vi "http_redirect.vi"(10 "Value":string, 11 "HTTP Request in in":T1) -> (3 "HTTP Request in out":T1)   [LabVIEW 2011]
uses:
  http_request_response.ctl
  http_request.ctl
  http_field.ctl
  http_response.ctl
  template_field.ctl
  template_field_type.ctl
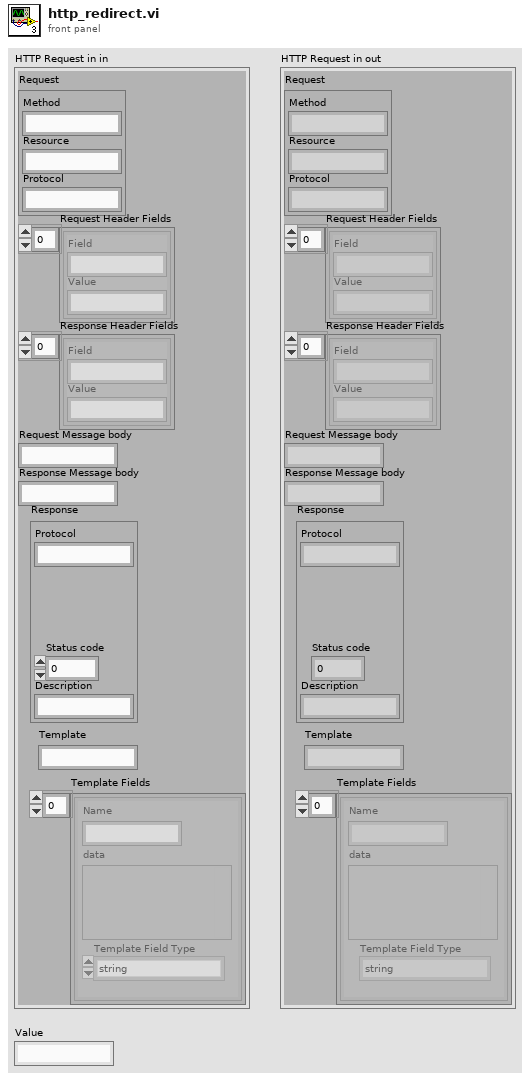
[diagram p1: front panel]
types:
  T1 = typedef "http_request_response.ctl" = cluster{"Request":T2, "Request Header Fields":T3[], "Response Header Fields":T3[], "Request Message body":string, "Response Message body":string, "Response":T4, "Template":string, "Template Fields":T5[]}
  T2 = typedef "http_request.ctl" = cluster{"Method":string, "Resource":string, "Protocol":string}
  T3 = typedef "http_field.ctl" = cluster{"Field":string, "Value":string}
  T4 = typedef "http_response.ctl" = cluster{"Protocol":string, "Status code":dbl, "Description":string}
  T5 = typedef "template_field.ctl" = cluster{"Name":string, "Template Field Type":T6, "data":variant}
  T6 = typedef "template_field_type.ctl" = enum16{"string", "string array", "number", "number array", "cluster", "cluster array"}
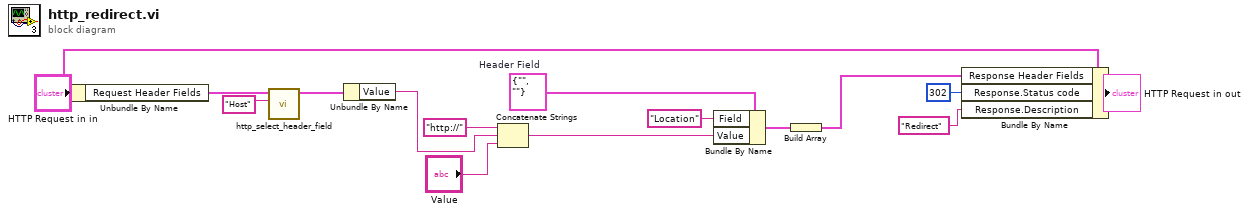
[diagram p0: block diagram]
diagram:
  w3 = T3 {"Field"="", "Value"=""}  # Header Field
  n1 = Unbundle By Name("HTTP Request in in") -> ("Request Header Fields"=w7:T3[])
  n2 = call "http_select_header_field.vi"("Name"="Host", "Request Header Fields"=w7) -> ("Header Field"=w9:T3)  [unwired: 8 in, 1 out]
  n3 = Unbundle By Name(w9) -> ("Value"=w10:string)
  n4 = Concatenate Strings("http://" ("string"), w10, "Value") -> (w12:string)
  n5 = Bundle By Name(cluster=w3, "Field"="Location", "Value"=w12) -> (w4:T3)
  n6 = Build Array(w4) -> (w2:T3[])
  n7 = Bundle By Name(cluster="HTTP Request in in", "Response Header Fields"=w2, "Response.Status code"=u16 302, "Response.Description"="Redirect") -> (→"HTTP Request in out":T1)
